vi "16-ParseTypeID.vi"(11 "BITS in":bool[](array[boolean])) -> (2 "TypeID":T1(ring), 3 "BITS out":bool[](array[boolean]))   [LabVIEW 2019, in "16.lvlib"]
uses:
  16.lvlib
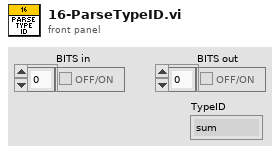
[diagram p1: front panel]
types:
  T1 = enum16{"sum", "product", "minimum", "maximum", "literal", "greater than", "less than", "equal to"}
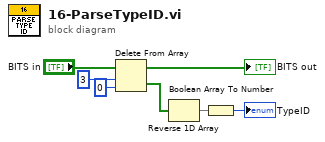
[diagram p0: block diagram]
diagram:
  n1 = Delete From Array(array="BITS in", length=3, index=0) -> (deleted portion=w4:bool[], array with subset deleted=→"BITS out":bool[])
  n2 = Reverse 1D Array(array=w4) -> (reversed array=w7:bool[])
  n3 = Boolean Array To Number(Boolean array=w7) -> (number=→"TypeID":u32)
